vi "Arm Controller.vi"(8 "error in":errorcluster) -> ()   [LabVIEW 2016]
doc: "This VI executes continuously carrying out the current operation and responding to updates or new operations. It will often contain the timing or control code that is difficult to place directly in TeleOp. This VI generally opens all sensors and motors and isolates the rest of the robot code from knowing how the operations are carried out."
uses:
  Arm Setpoints.ctl
  Arm Operations.ctl
  <vilib>/Rock Robotics/WPI/SafetyOutput/WPI_SafetyOutputConfigMenu.ctl
  <vilib>/Rock Robotics/WPI/Utilities/WPI_GetSetVariantRefNum.vi
  <vilib>/Rock Robotics/Network Tables/NT Write Boolean.vi
panel:
  out "Setpoints":T1(graph)
  out "Current\nCmd":string
  # "Tip: It may be helpful to observe inputs and sensor values.\nYou may also want to display tuning or debugging controls."
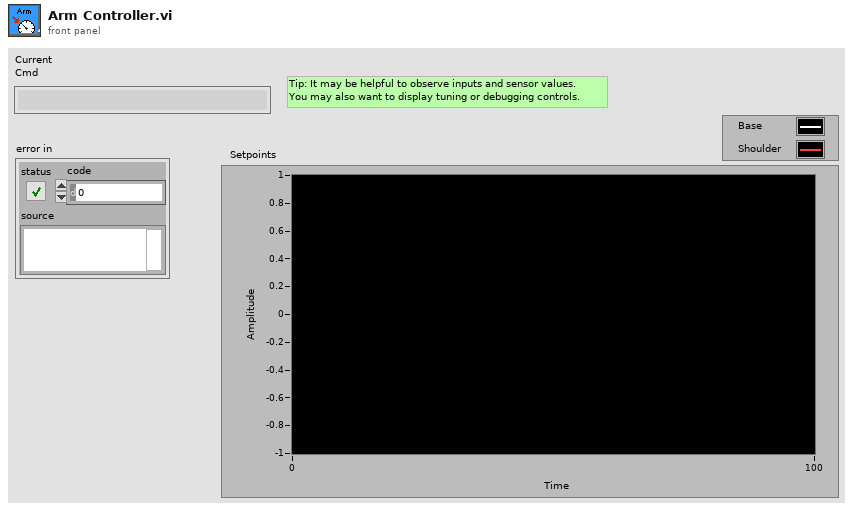
[diagram p1: front panel]
types:
  T1 = cluster{"Left Setpoint":dbl, "Right Setpoint":dbl}
  T2 = typedef "WPI_SafetyOutputConfigMenu.ctl" = enum16{"Enable", "Disable"}
  T3 = typedef "Arm Setpoints.ctl" = cluster{"Operation":T4, "Duration":dbl, "Base Setpoint":dbl, "Shoulder Setpoint":dbl, "Gripper":dbl}
  T4 = typedef "Arm Operations.ctl" = enum16{"Reserve", "Read Current", "Immediate", "Close Gripper", "Open Gripper"}
  T5 = typedef "WPI_RobotDriveDevRef.ctl" = cluster{"DevStatus":errorcluster, "Motors[]":T6[], "Square Inputs":bool, "Max Output":dbl}
  T6 = typedef "WPI_MotorControlDeviceRef.ctl" = cluster{"DeviceStatus":errorcluster, "Type":T7, "PWM":cluster{"PWM Channel":T8, "DeadBand":T9}, "CAN":cluster{"Device Number":u8, "SetOutput VI Ref":variant, "GetOutput VI Ref":variant, "Enable VI Ref":variant, "Disable VI Ref":variant, "Data":variant}, "Invert":bool}
  T7 = typedef "WPI_MotorControlType.ctl" = enum16{"PWM", "CAN"}
  T8 = typedef "FPGA_DIOPWMChannel.ctl" = enum8{"PWM 0", "PWM 1", "PWM 2", "PWM 3", "PWM 4", "PWM 5", "PWM 6", "PWM 7", "PWM 8", "PWM 9", "PWM MXP 0", "PWM MXP 1", "PWM MXP 2", "PWM MXP 3", "PWM MXP 4", "PWM MXP 5", "PWM MXP 6", "PWM MXP 7", "PWM MXP 8", "PWM MXP 9", "Invalid"}
  T9 = typedef "WPI_PWMDeadband.ctl" = cluster{"Name":string, "maxPositivePwm":i32, "minPositivePwm":i32, "centerPwm":i32, "maxNegativePwm":i32, "minNegativePwm":i32, "angularRange":u16}
  T10 = typedef "Command Status Info.ctl" = cluster{"Name":string, "Status":T11, "notifier out":T12}
  T11 = typedef "Completion Status.ctl" = enum16{"Successful", "Aborted", "Incomplete"}
  T12 = typedef "Completion Notifier.ctl" = refnum<notifier>
  T13 = cluster{"Default Command":T3, "Command Timing":cluster{"Start Time (ms)":u32, "Iterations":i32}, "Command Arguments":cluster{"Command Info":T10, "Description":string, "Default Command":T3, "notifier out":refnum<notifier>, "Subsystem Name":string}}
  T14 = cluster{"Base Setpoint":dbl, "Shoulder Setpoint":dbl}
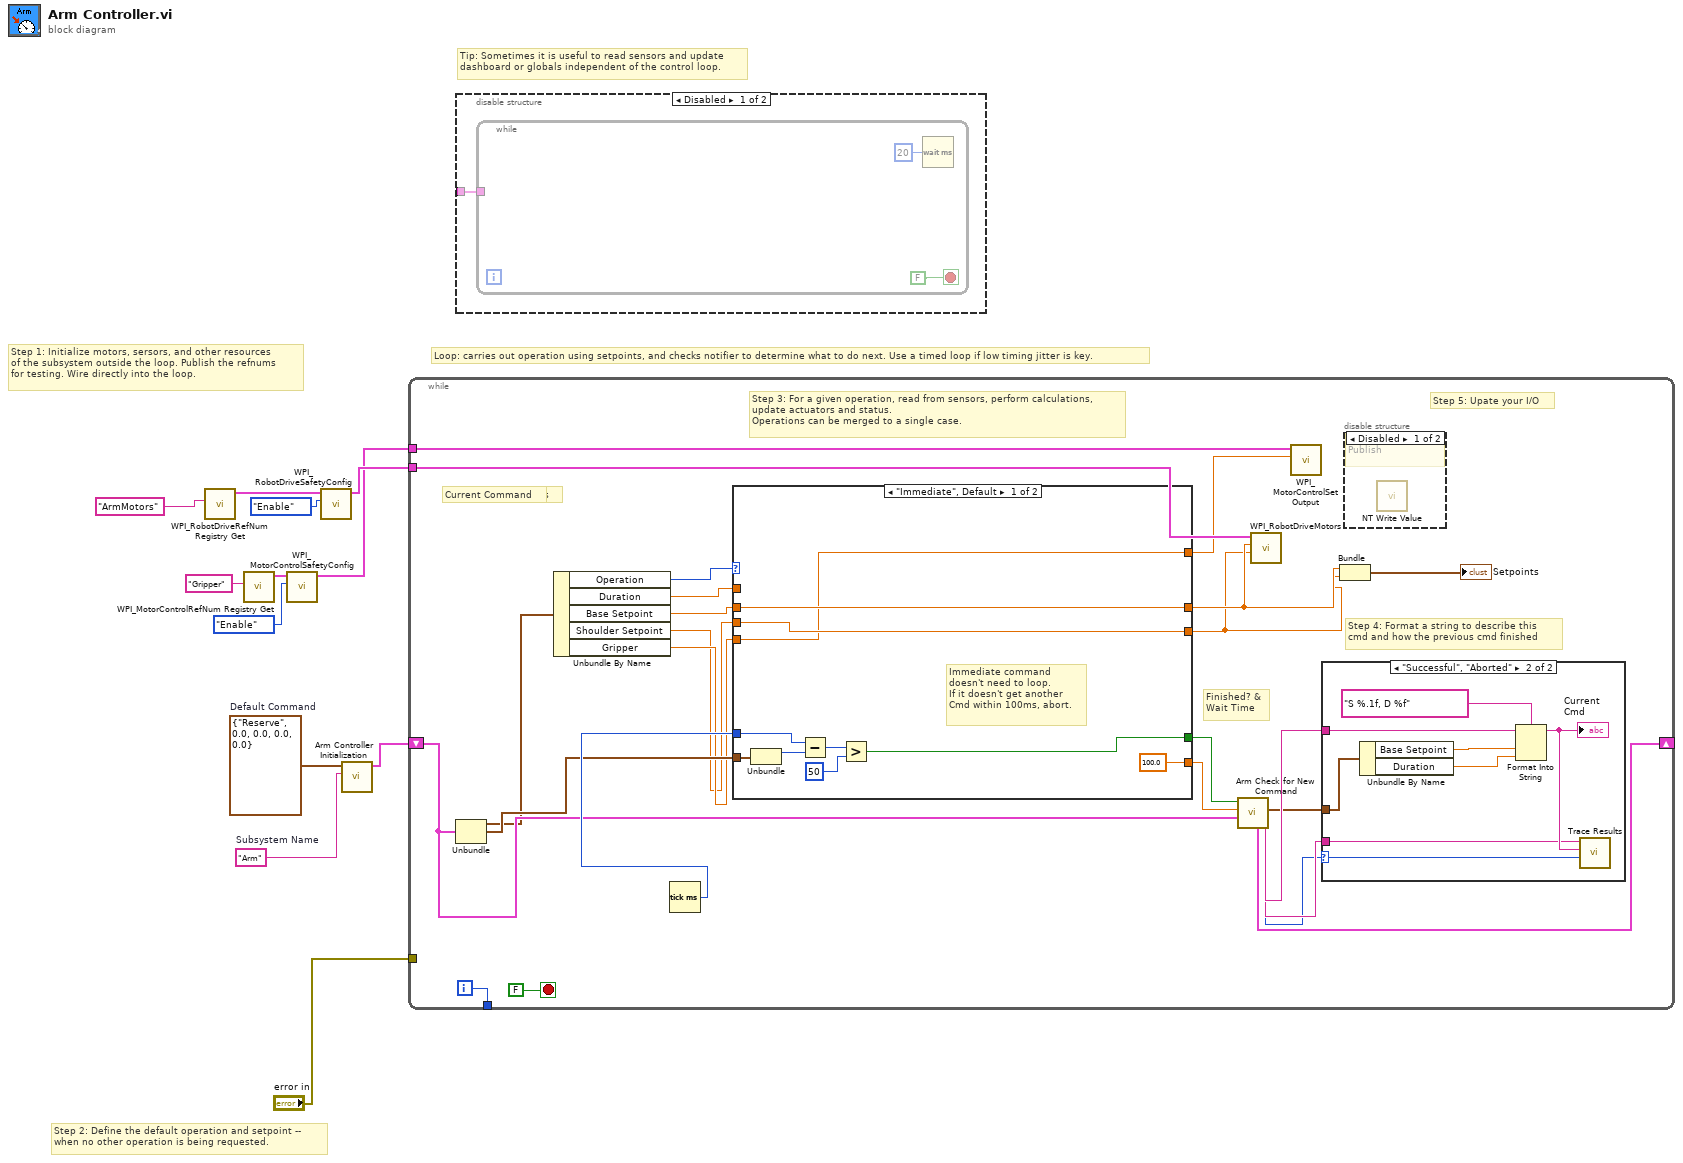
[diagram p0: block diagram]
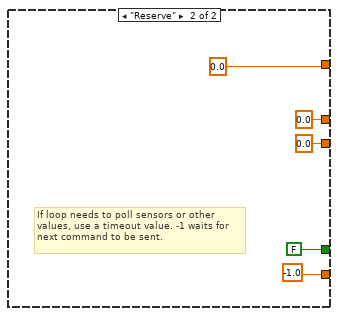
[diagram p5: hidden frame]
diagram:
  w9 = T3 {"Operation"=enum."Reserve", "Duration"=0.0, "Base Setpoint"=0.0, "Shoulder Setpoint"=0.0, "Gripper"=0.0}  # Default Command
  w10 = "Arm"  # Subsystem Name
  # "Tip: Sometimes it is useful to read sensors and update\ndashboard or globals independent of the control loop."
  # "Step 2: Define the default operation and setpoint --\nwhen no other operation is being requested."
  # "Step 1: Initialize motors, sersors, and other resources\nof the subsystem outside the loop. Publish the refnums\nfor testing. Wire directly into the loop."
  # "Loop: carries out operation using setpoints, and checks notifier to determine what to do next. Use a timed loop if low timing jitter is key."
  n1 = call <vilib>:"WPI_RobotDriveRefNum Registry Get.vi"("refnum name"="ArmMotors") -> ("RobotDriveDevRef"=w7:T5)  [unwired: 9 in, 1 out]
  n2 = call <vilib>:"WPI_MotorControlRefNum Registry Get.vi"("refnum name"="Gripper") -> ("MotorControlDevRef"=w2:T6)  [unwired: 9 in, 1 out]
  n3 = call <vilib>:"WPI_MotorControlSafetyConfig.vi"("mode"=WPI_SafetyOutputConfigMenu."Enable", "MotorControlDevRef"=w2) -> ("MotorControlDevRef"=w1:T6)  [unwired: 8 in, 1 out]
  n4 = call <vilib>:"WPI_RobotDriveSafetyConfig.vi"("mode"=WPI_SafetyOutputConfigMenu."Enable", "RobotDriveDevRef"=w7) -> ("RobotDriveDevRef"=w5:T5)  [unwired: 8 in, 1 out]
  n5 = call "Arm Controller Initialization.vi"("Subsystem Name"=w10, "Default Command"=w9) -> ("Command Info"=w11:T13)  [unwired: 9 in]
  n6 = while {
    shift-right: [w31] -> _
    shift-left: w11 -> [w32]
    tunnel: [w35] -> _
    tunnel: "error in" -> [_]
    tunnel: w5 -> [w24]
    tunnel: w1 -> [w20]
    i -> [w35]
    stop <- FALSE stop-if-true
    # "Step 5: Upate your I/O"
    # "Step 4: Format a string to describe this\ncmd and how the previous cmd finished"
    # "Current Command"
    # "Access Cmd setpoints"
    # "Finished? &\nWait Time"
    # "Step 3: For a given operation, read from sensors, perform calculations,\nupdate actuators and status.\nOperations can be merged to a single case."
    n7 = Unbundle(w32) -> ("Default Command"=w18:T3, "Command Timing"=w33:cluster{"Start Time (ms)":u32, "Iterations":i32})  [unwired: 1 out]
    n8 = Unbundle By Name(w18) -> ("Operation"=w13:T4, "Duration"=w14:dbl, "Base Setpoint"=w15:dbl, "Shoulder Setpoint"=w16:dbl, "Gripper"=w17:dbl)
    n9 = Tick Count (ms)() -> (millisecond timer value=w34:u32)
    n10 = case shown="\"Immediate\", Default" w13 {
      tunnel: [100.0 -1.0] -> w29
      tunnel: [w48 FALSE ("ignore previous (F)")] -> w30
      tunnel: w33 -> [w50 _]
      tunnel: w14 -> [_ _]
      tunnel: w34 -> [w49 _]
      tunnel: w15 -> [w47 _]
      tunnel: [w47 0.0 ("Base Setpoint")] -> w23
      tunnel: w16 -> [w46 _]
      tunnel: [w46 0.0 ("Shoulder Setpoint")] -> w22
      tunnel: [w45 0.0 ("Base Setpoint")] -> w19
      tunnel: w17 -> [w45 _]
      frame "Immediate", Default {
        # "Immediate command\ndoesn't need to loop.\nIf it doesn't get another\nCmd within 100ms, abort."
        n11 = Unbundle(w50) -> ("Start Time (ms)"=w53:u32)  [unwired: 1 out]
        n12 = Subtract(x=w49, y=w53) -> (x-y=w52:u32)
        n13 = Greater?(x=w52, y=u8 50 ("Left Motor")) -> (0:w48:bool)
      }
      frame "Reserve" {
        # "If loop needs to poll sensors or other\nvalues, use a timeout value. -1 waits for\nnext command to be sent."
      }
    }
    n14 = call "Arm Check for New Command.vi"("Current Command"=w32, "Wait time (ms)"=w29, "Finished?"=w30) -> ("Completion"=w25:T11, "Subsystem Name"=w26:string, "Current Command"=w27:T3, "Initial Trace String"=w28:string, "NextCommand"=w31:T13)  [unwired: 4 in]
    n15 = call <vilib>:"WPI_RobotDriveMotors.vi"("RightSpeed"=w22, "LeftSpeed"=w23, "RobotDriveDevRef"=w24) -> ()  [unwired: 6 in, 3 out]
    n16 = call <vilib>:"WPI_MotorControlSetOutput.vi"("Output"=w19, "MotorControlDevRef"=w20) -> ()  [unwired: 7 in, 3 out]
    n17 = case shown="\"Successful\", \"Aborted\"" w25 {
      selector: w25 -> [_ w44]
      tunnel: w28 -> [_ w40]
      tunnel: w27 -> [_ w41]
      tunnel: w26 -> [_ w37]
      frame "Incomplete", Default {
        # "Continuing current command"
      }
      frame "Successful", "Aborted" {
        # "Report and setup for next command"
        n18 = Unbundle By Name(w41) -> ("Base Setpoint"=w43:dbl, "Duration"=w38:dbl)
        n19 = Format Into String(format string="S %.1f, D %f", initial string=w40, w43, w38) -> (resulting string=w39:string)  [unwired: 1 in, 1 out]
        "Current\nCmd" <- w39
        n20 = call <vilib>:"Trace Results.vi"("Status of previous command"=w44, "Description"=w39, "Subsystem"=w37) -> ()  [unwired: 9 in]
      }
    }
    n21 = Bundle("Base Setpoint"=w23, "Shoulder Setpoint"=w22) -> (→"Setpoints":T14)  [unwired: 1 in]
    n22 = disable-structure shown="Disabled" {
      frame Disabled {
        # "Publish"
        n23 = call-poly <vilib>:"NT Write Value.vi"() -> ()  [unwired: 11 in, 1 out]
      }
      frame Enabled {
      }
    }
  }
  n24 = disable-structure shown="Disabled" {
    disable-tunnel: _ -> [w60 _]
    frame Disabled {
      n25 = while {
        tunnel: w60 -> [_]
        stop <- FALSE stop-if-true
        n26 = Wait (ms)(milliseconds to wait=u32 20) -> ()  [unwired: 1 out]
      }
    }
    frame Enabled {
    }
  }
